vi "KT2_Temperature.vi"() -> (3 "Temperature":dbl)   [LabVIEW 2018]
doc: "This VI reads the temperature values every second"
uses:
  KT2/Paskevits_Vladislav_gbl1.vi
  KT2/Paskevits_Vladislav_gbl.vi
panel:
  out "Waveform Chart":dbl[](graph)
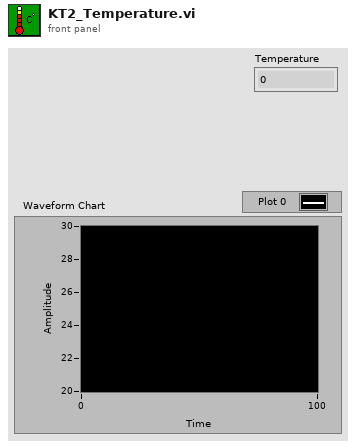
[diagram p1: front panel]
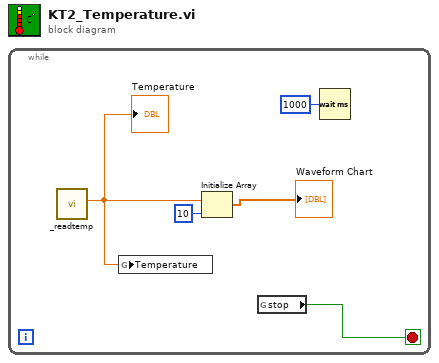
[diagram p0: block diagram]
diagram:
  n1 = while {
    stop <- w4 stop-if-true
    n2 = call "_readtemp.vi"() -> ("Temperature"=w2:dbl)  [unwired: 10 in, 1 out]
    "Temperature" <- w2
    n3 = global write "Paskevits_Vladislav_gbl1.vi" "Temperature"(w2) -> ()
    n4 = Initialize Array(w2, 10 ("dimension size")) -> (→"Waveform Chart":dbl[])
    n5 = global read "Paskevits_Vladislav_gbl.vi" "stop"() -> (w4:bool)
    n6 = Wait (ms)(milliseconds to wait=u32 1000) -> ()  [unwired: 1 out]
  }
